vi "Test_WriteValue_InvalidType_Error.vi"(8 "error in (no error)":errorcluster, 11 "TestCase in":refnum<class "TestTerminalValueBinding.lvclass">) -> (0 "error out":errorcluster, 3 "TestCase out":refnum<class "TestTerminalValueBinding.lvclass">)   [LabVIEW 2017, in "TestTerminalValueBinding.lvclass"]
uses:
  TestTerminalValueBinding.lvclass
  Source/Concrete/TerminalValueBinding/TerminalValueBinding.lvclass
  C:/Git/composed-transport/Source/ITransport/ITransport.lvclass
  Source/ITransport/ITransport.lvclass
panel:
  out "Return Error":errorcluster
  in  "Not a Numeric":bool
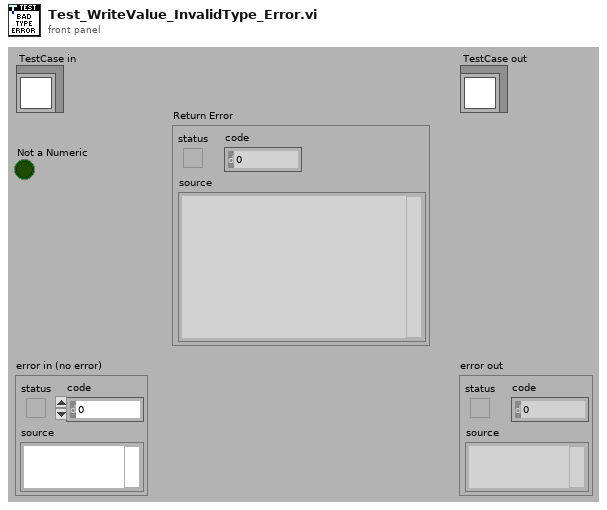
[diagram p1: front panel]
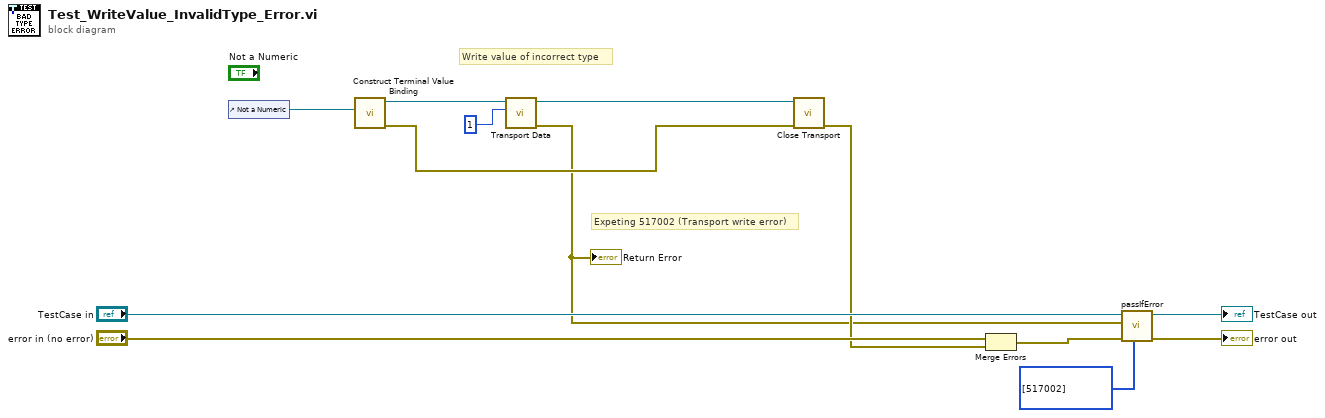
[diagram p0: block diagram]
diagram:
  # "Expeting 517002 (Transport write error)"
  # "Write value of incorrect type"
  n1 = control-ref of="Not a Numeric"() -> (w5:refnum<vi>)
  n2 = call "Construct Terminal Value Binding.vi"("Ctl Refnum"=w5) -> ("error out"=w3:errorcluster, "TerminalValueBinding Out"=w9:refnum<class "TerminalValueBinding.lvclass">)  [unwired: 9 in]
  n3 = call "Transport Data.vi"("Value"=1, "ITransport in"=w9) -> ("error out"=w2:errorcluster, "ITransport out"=w6:refnum<class "TerminalValueBinding.lvclass">)  [unwired: 8 in]
  "Return Error" <- w2
  n4 = call-dynamic "Close Transport.vi"("error in (no error)"=w3, "ITransport in"=w6) -> ("error out"=w4:errorcluster)  [unwired: 9 in]
  n5 = Merge Errors("error in (no error)", w4) -> (w8:errorcluster)
  n6 = call-dynamic "passIfError.vi"("passing error codes (default = any error code)"=i32[] [517002], "error in (no error)"=w8, "error"=w2, "TestCase in"="TestCase in") -> ("error out"=→"error out":errorcluster, "TestCase out"=→"TestCase out":refnum<class "TestTerminalValueBinding.lvclass">)  [unwired: 6 in]
